vi "Close.vi"(8 "error in (no error)":errorcluster, 10 "Msg in":T1, 11 "MagSpec_Bella in":refnum<class "MagSpec_Bella.lvclass">) -> (0 "error out":errorcluster, 1 "new command":string, 2 "Msg out":T1, 3 "MagSpec_Bella out":refnum<class "MagSpec_Bella.lvclass">)   [LabVIEW 2013, in "MagSpec_Bella.lvclass"]
uses:
  MagSpec_Bella.lvclass
  BaseDriver/DriverMsg.ctl
  BaseDriver/BaseDriver.lvclass
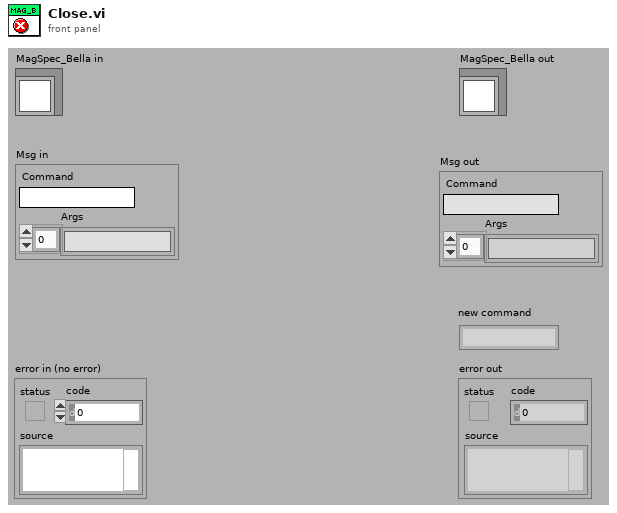
[diagram p1: front panel]
types:
  T1 = typedef "DriverMsg.ctl" = cluster{"Command":string, "Args":string[]}
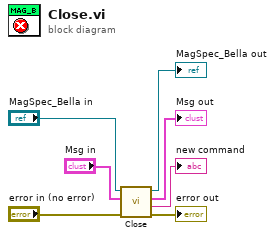
[diagram p0: block diagram]
diagram:
  n1 = call-parent "Close.vi"("error in (no error)"="error in (no error)", "Msg in"="Msg in", "BaseDriver in"="MagSpec_Bella in") -> ("error out"=→"error out":errorcluster, "new command"=→"new command":string, "Msg out"=→"Msg out":T1, "BaseDriver out"=→"MagSpec_Bella out":refnum<class "MagSpec_Bella.lvclass">)  [unwired: 5 in]
